vi "MGI B-Spline.vi"(1 "x":dbl, 2 "Knot Multiplicities":i32[](array[numeric]), 3 "Knots":dbl[](array[numeric]), 4 "Control Points[][]":dbl[][](array[numeric])) -> (0 "S(x)":dbl[](array[numeric]))   [LabVIEW 2016]
doc: "Calculate a B-Spline curve value using the de Boor algorithm. Input is formatted for compatibility with a STEP file (ISO-10303).\n\nFreeware from Moore Good Ideas, www.mooregoodideas.com. Do not remove this line."
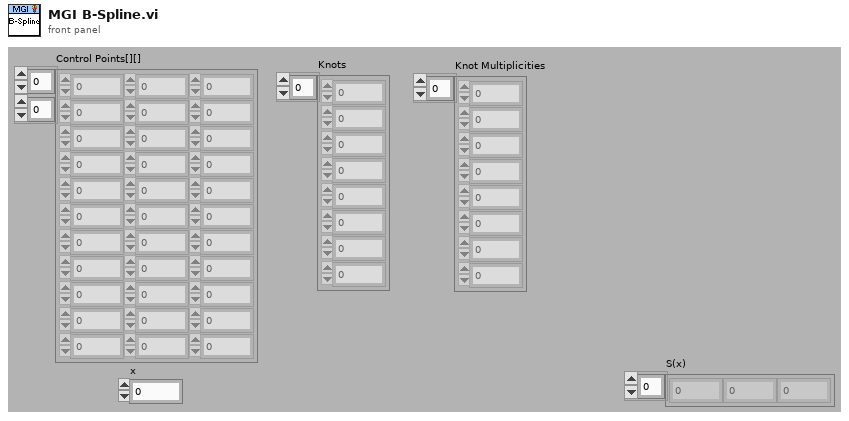
[diagram p1: front panel]
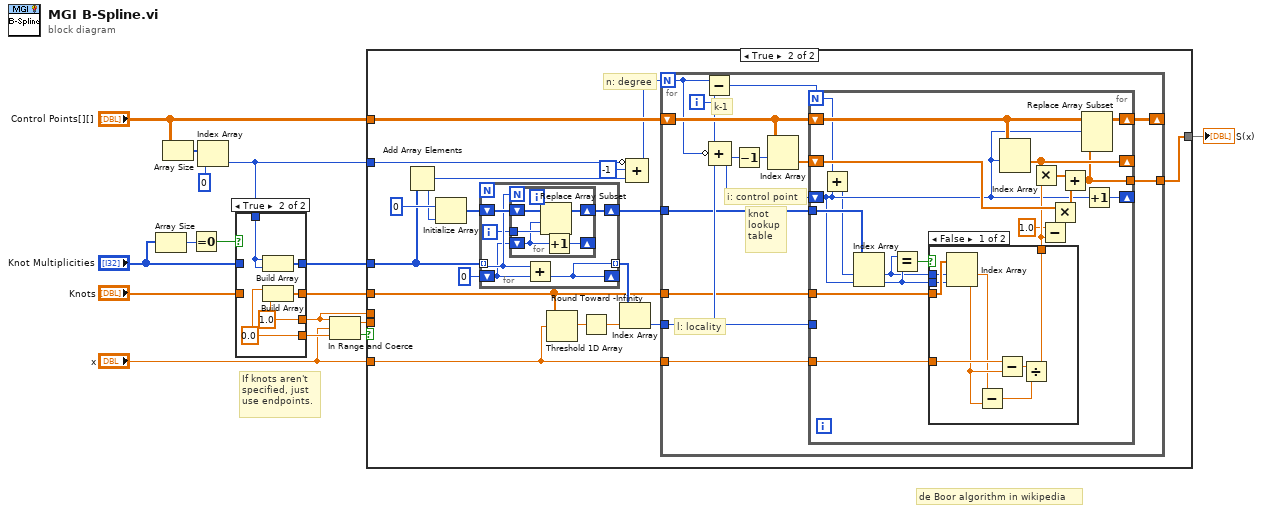
[diagram p0: block diagram]
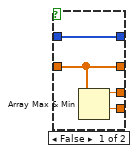
[diagram p2: hidden frame]
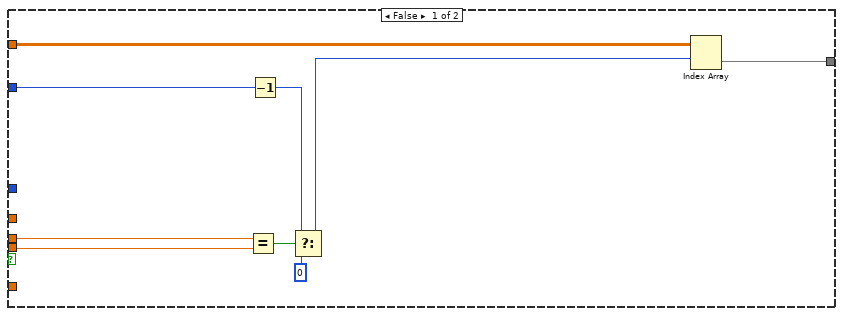
[diagram p3: hidden frame]
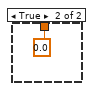
[diagram p4: hidden frame]
diagram:
  # "If knots aren't\nspecified, just\nuse endpoints."
  # "de Boor algorithm in wikipedia"
  n1 = Array Size(array="Knot Multiplicities") -> (size(s)=w2:i32)
  n2 = Array Size(array="Control Points[][]") -> (size(s)=w8:i32[])
  n3 = Equal To 0?(x=w2) -> (x = 0?=w1:bool)
  n4 = Index Array(array=w8, index=0) -> (element=w4:i32)
  n5 = case shown="True" w1 {
    tunnel: "Knots" -> [w17 _]
    tunnel: [w20 w24] -> w15
    tunnel: [w19 w25] -> w11
    tunnel: "Knot Multiplicities" -> [w18 _]
    tunnel: [w18 w21] -> w6
    tunnel: [w17 w23] -> w5
    tunnel: w4 -> [_ w22]
    frame False {
      n6 = Array Max & Min(array=w17) -> (max value=w19:dbl, min value=w20:dbl)  [unwired: 2 out]
    }
    frame True {
      w24 = 0.0
      w25 = 1.0
      n7 = Build Array(w22, w22) -> (w21:i32[])
      n8 = Build Array(w24, w25) -> (w23:dbl[])
    }
  }
  n9 = In Range and Coerce(upper limit=w11, x="x", lower limit=w15) -> (coerced(x)=w12:dbl, In Range?=w13:bool)
  n10 = case shown="True" w13 {
    tunnel: w5 -> [_ w36]
    tunnel: "x" -> [_ w44]
    tunnel: w12 -> [w34 _]
    tunnel: w11 -> [w33 _]
    tunnel: "Control Points[][]" -> [w32 w49]
    tunnel: [w31 w35] -> w10
    tunnel: w4 -> [w30 w51]
    tunnel: w6 -> [_ w41]
    frame False {
      n11 = Equal?(x=w33, y=w34) -> (x = y?=w29:bool)
      n12 = Decrement(x=w30) -> (x-1=w28:i32)
      n13 = Select(t=w28, s=w29, f=0) -> (s? t:f=w26:i32)
      n14 = Index Array(array=w32, index (row)=w26) -> (element=w31:dbl[])  [unwired: 1 in]
    }
    frame True {
      # "n: degree"
      n15 = Add Array Elements(numeric array=w41) -> (sum=w40:i32)
      n16 = Initialize Array(0 ("element"), w40) -> (w43:i32[])
      n17 = for {
        tunnel: w41 -> [w54] mode=indexing
        shift-right: [w57] -> _
        shift-left: 0 -> [w52]
        tunnel: [w57] -> w39 mode=indexing
        shift-right: [w55] -> w37
        shift-left: w43 -> [w56]
        i -> [w53]
        n18 = for {
          N: w54 -> [_]
          shift-right: [w61] -> w55
          shift-left: w56 -> [w62]
          tunnel: w53 -> [w60]
          shift-right: [w58] -> _
          shift-left: w52 -> [w59]
          n19 = Replace Array Subset(array=w62, new element=w60, index=w59) -> (w61:i32[])
          n20 = Increment(x=w59) -> (x+1=w58:i32)
        }
        n21 = Add(x=w54, y=w52) -> (x+y=w57:i32)
      }
      n22 = Threshold 1D Array(2:w44, 3:w36) -> (0:w48:dbl)  [unwired: 1 out]
      n23 = Round Toward -Infinity(1:w48) -> (0:w46:dbl)
      n24 = Index Array(array=w39, index=w46) -> (element=w45:i32)
      n25 = Compound Arithmetic op=ADD(invert w51, -1 ("value"), w40) -> (w47:i32)
      n26 = for {
        N: w47 -> [w69]
        shift-right: [w75] -> _
        shift-left: w49 -> [w72]
        tunnel: w45 -> [w71]
        tunnel: w44 -> [w66]
        tunnel: w37 -> [w65]
        tunnel: w36 -> [w64]
        tunnel: [w63] -> w35
        i -> [w70]
        # "i: control point"
        # "knot\nlookup\ntable"
        # "l: locality"
        # "k-1"
        n27 = Subtract(x=w69, y=w70) -> (x-y=w74:i32)
        n28 = Compound Arithmetic op=ADD(w70, invert w69, w71) -> (w68:i32)
        n29 = Decrement(x=w68) -> (x-1=w67:i32)
        n30 = Index Array(array=w72, index (row)=w67) -> (element=w73:dbl[])  [unwired: 1 in]
        n31 = for {
          N: w74 -> [w80]
          shift-right: [w94] -> w75
          shift-left: w72 -> [w95]
          tunnel: w71 -> [_]
          shift-right: [w91] -> _
          shift-left: w73 -> [w92]
          shift-right: [w93] -> _
          shift-left: w68 -> [w81]
          tunnel: w66 -> [w88]
          tunnel: w65 -> [w87]
          tunnel: w64 -> [w86]
          tunnel: [w82] -> w63
          n32 = Add(x=w80, y=w81) -> (x+y=w79:i32)
          n33 = Index Array(array=w87, index #1=w79, index #2=w81) -> (element #1=w77:i32, element #2=w78:i32)
          n34 = Equal?(x=w77, y=w78) -> (x = y?=w76:bool)
          n35 = case shown="False" w76 {
            tunnel: w88 -> [w104 _]
            tunnel: w86 -> [w103 _]
            tunnel: [w99 0.0] -> w84
            tunnel: w78 -> [w97 _]
            tunnel: w77 -> [w96 _]
            frame False {
              n36 = Index Array(array=w103, index #1=w96, index #2=w97) -> (element #1=w98:dbl, element #2=w101:dbl)
              n37 = Subtract(x=w98, y=w101) -> (x-y=w100:dbl)
              n38 = Subtract(x=w104, y=w101) -> (x-y=w102:dbl)
              n39 = Divide(x=w102, y=w100) -> (x/y=w99:dbl)
            }
            frame True {
            }
          }
          n40 = Index Array(array=w95, index (row)=w81) -> (element=w91:dbl[])  [unwired: 1 in]
          n41 = Multiply(x=w91, y=w84) -> (x*y=w90:dbl[])
          n42 = Subtract(x=1.0, y=w84) -> (x-y=w85:dbl)
          n43 = Multiply(x=w92, y=w85) -> (x*y=w89:dbl[])
          n44 = Add(x=w90, y=w89) -> (x+y=w82:dbl[])
          n45 = Replace Array Subset(array=w95, new element=w82, index (row)=w81) -> (w94:dbl[][])  [unwired: 1 in]
          n46 = Increment(x=w81) -> (x+1=w93:i32)
        }
      }
    }
  }
  "S(x)" <- w10
